vi "3. In CSM API parameters.vi"() -> ()   [LabVIEW 2017]
doc: "## Persisting CSM API Parameters (3. In CSM API parameters.vi)\n\n### Overview\n\nDemonstrates how to use the CSM INI Variable Support feature to persist parameter information in an INI configuration file.\n\n### Introduction\n\nThis example shows how to persist parameter information in an INI configuration file using CSM INI Variable Support API, primarily through `Convert API String to Cluster(Default in Session).vim` or `Convert API String to Cluster(Default in Key).vim`. They function identically to their counterparts in CSM API String Support but add the functionality of reading INI configuration files.\n\nData sources may include: information sent via message parameters, parameters in the configuration file, or default constant parameters provided at design time. They have a clear priority hierarchy: CSM API Parameters > Configuration File Parameters > Default Constant Parameters.\n\n**Notes:**\n\n- During initialization, explicitly sent parameters have the highest priority.\n- If no parameters are sent, parameters from the configuration file are used.\n- In the absence of configuration file parameters, default constant parameters are applied.\n- Parameters can be partially specified. Missing values are automatically filled using configuration information from the next priority level.\n\n### Steps\n\n- Step1: Generate a temporary INI file and load it using `CSM - Load Configuration Variables From File.vi`.\n\n- Step2: Simulate a CSM module named \"network\" using a standard loop.\n\n- Step3: Assume the passed parameter is \"ip:11.22.33.44\". This information has the highest priority and overrides the configuration in the INI file.\n\n - Step3.1: `Convert API String to Cluster(Default in Session).vim` conversion loads the key with the same name from the section. The IP information is loaded from the parameter. The port is not provided in the parameter, but port is defined as 8080 in \"network\". So the final cluster port is 8080.\n - Step3.2: `Convert API String to Cluster(Default in Session).vim` conversion loads configuration from the given section/key. The IP information is loaded from the parameter. The port is not provided in the parameter, but port is defined as 8081 in network.address1. Thus the final cluster port is 8081.\n\n- Step4: Assume the passed parameter is empty `\"\"`, equivalent to providing no parameter. In this case, the configuration from the file is prioritized.\n\n - Step4.1: `Convert API String to Cluster(Default in Session).vim` conversion loads the key with the same name from the section. The IP information uses network.ip, resulting in IP: 10.144.41.41. The port uses network.port, resulting in 8080.\n - Step4.2: `Convert API String to Cluster(Default in Session).vim` conversion loads configuration from the given section/key. Configuration is loaded from network.address1, resulting in IP:10.144.42.42 and port:8081.\n\n- Step5: Assume the passed parameter is empty `\"\"`, equivalent to providing no parameter. The corresponding configuration is not defined in the INI configuration file. In this case, default constant parameters are used.\n\n - Step5.1: `Convert API String to Cluster(Default in Session).vim` conversion. The \"non-existing module\" section does not exist, so the provided reference data is used, resulting in IP:127.0.0.1 and port:80.\n - Step5.2: `Convert API String to Cluster(Default in Session).vim` conversion. Load configuration from the given section/key, but neither exists. The provided reference data is used, resulting in IP:127.0.0.1 and port:80."
uses:
  1656162b-afee-422c-bd32-e5dc0ed47e9c.vi
  10c63860-64da-4a50-8590-83a789bccc1b.vi
  b8deca2c-73dd-4ae4-bcf2-ddb52dad5ebe.vi
  2f71b960-401c-4d78-a3a0-f07855567af6.vi
  000051f1-0e83-4b30-8694-14c2d9f7239e.vi
  0af89d8b-3541-4ee1-9e23-b806c46e6636.vi
  1656162b-afee-422c-bd32-e5dc0ed47e9c.vi/70cf541c-689a-4909-ae73-497058dc5e15.vi
  1656162b-afee-422c-bd32-e5dc0ed47e9c.vi/8441470c-f7c2-4ba6-a00e-bb382131ed64.vi
  10c63860-64da-4a50-8590-83a789bccc1b.vi/70cf541c-689a-4909-ae73-497058dc5e15.vi
  10c63860-64da-4a50-8590-83a789bccc1b.vi/9171d6c3-d5ea-4572-92dd-59f7e0660fdf.vi
  b8deca2c-73dd-4ae4-bcf2-ddb52dad5ebe.vi/70cf541c-689a-4909-ae73-497058dc5e15.vi
  b8deca2c-73dd-4ae4-bcf2-ddb52dad5ebe.vi/9171d6c3-d5ea-4572-92dd-59f7e0660fdf.vi
  2f71b960-401c-4d78-a3a0-f07855567af6.vi/70cf541c-689a-4909-ae73-497058dc5e15.vi
  2f71b960-401c-4d78-a3a0-f07855567af6.vi/8441470c-f7c2-4ba6-a00e-bb382131ed64.vi
  000051f1-0e83-4b30-8694-14c2d9f7239e.vi/70cf541c-689a-4909-ae73-497058dc5e15.vi
  000051f1-0e83-4b30-8694-14c2d9f7239e.vi/8441470c-f7c2-4ba6-a00e-bb382131ed64.vi
  0af89d8b-3541-4ee1-9e23-b806c46e6636.vi/70cf541c-689a-4909-ae73-497058dc5e15.vi
  0af89d8b-3541-4ee1-9e23-b806c46e6636.vi/9171d6c3-d5ea-4572-92dd-59f7e0660fdf.vi
  1656162b-afee-422c-bd32-e5dc0ed47e9c.vi/8441470c-f7c2-4ba6-a00e-bb382131ed64.vi/99de0c97-112a-4c86-9094-c187659127e1.vi
  <userlib>/_NEVSTOP/Communicable State Machine(CSM)/Utility/Build Error Cluster.vi
  <userlib>/_NEVSTOP/Communicable State Machine(CSM)/addons/API-String-Arugments-Support/_Support/Concatenate Strings If not Empty_csm.vi
  INI-Static-Variable-Support/_Support/FlagInstance-CSMINIVariable.vi
  2f71b960-401c-4d78-a3a0-f07855567af6.vi/8441470c-f7c2-4ba6-a00e-bb382131ed64.vi/99de0c97-112a-4c86-9094-c187659127e1.vi
  000051f1-0e83-4b30-8694-14c2d9f7239e.vi/8441470c-f7c2-4ba6-a00e-bb382131ed64.vi/99de0c97-112a-4c86-9094-c187659127e1.vi
  <userlib>/_NEVSTOP/Communicable State Machine(CSM)/_Support/ChangeFlag/ChangeFlag-Read.vi
  <userlib>/_NEVSTOP/Communicable State Machine(CSM)/_Support/ChangeFlag/ChangeFlagDB.vi
  INI-Static-Variable-Support/_Support/CSM - Read INI String.vi
  INI-Static-Variable-Support/_Support/Populate String with INI Variable.vi
  <userlib>/_NEVSTOP/Communicable State Machine(CSM)/addons/API-String-Arugments-Support/_Support/Convert API String Arguments to Data(variant).vi
  <vilib>/Utility/Data Type/Get Type Information.vi
  <userlib>/_NEVSTOP/Communicable State Machine(CSM)/addons/API-String-Arugments-Support/_Support/Data To SingleElementsArray_csm.vi
  <userlib>/_NEVSTOP/Communicable State Machine(CSM)/addons/API-String-Arugments-Support/_Support/Data To API String Arguments.vi
  INI-Static-Variable-Support/_Support/Parse Used Session and Name.vi
  INI-Static-Variable-Support/_Support/INI-FGV(lvlibp).vi
  <userlib>/_NEVSTOP/Communicable State Machine(CSM)/addons/API-String-Arugments-Support/_Support/SingleElementsArray To Data_csm.vi
  INI-Static-Variable-Support/INI-Static-Variable-Support.lvlib
panel:
  out "case1:(load from section) use default value of constant":cluster{"ip":string, "port":i32}={"ip"="127.0.0.1", "port"=80}
  out "case1:(load from key) use default value of constant":cluster{"ip":string, "port":i32}={"ip"="127.0.0.1", "port"=80}
  out "case2:(load from section) no argument, use config":cluster{"ip":string, "port":i32}={"ip"="10.144.41.41", "port"=8080}
  out "case2:(load from key) no argument, use config":cluster{"ip":string, "port":i32}={"ip"="10.144.42.42", "port"=8081}
  out "case3:(load from key) use argument value":cluster{"ip":string, "port":i32}={"ip"="11.22.33.44", "port"=8081}
  out "case3:(load from section) use argument value":cluster{"ip":string, "port":i32}={"ip"="11.22.33.44", "port"=8080}
  # "#CSM-Example overview\n\nDemonstrates how to use the CSM INI Variable Support feature to persist parameter information in an INI configuration file."
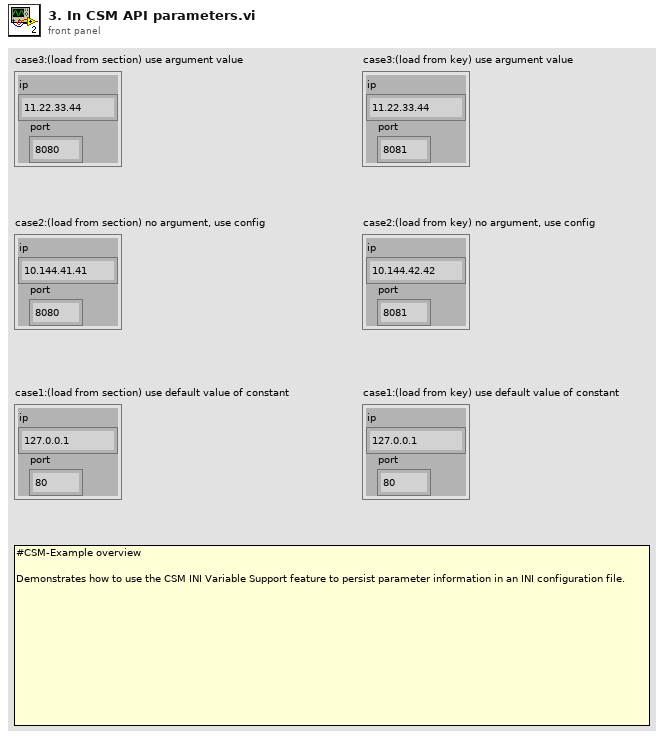
[diagram p1: front panel]
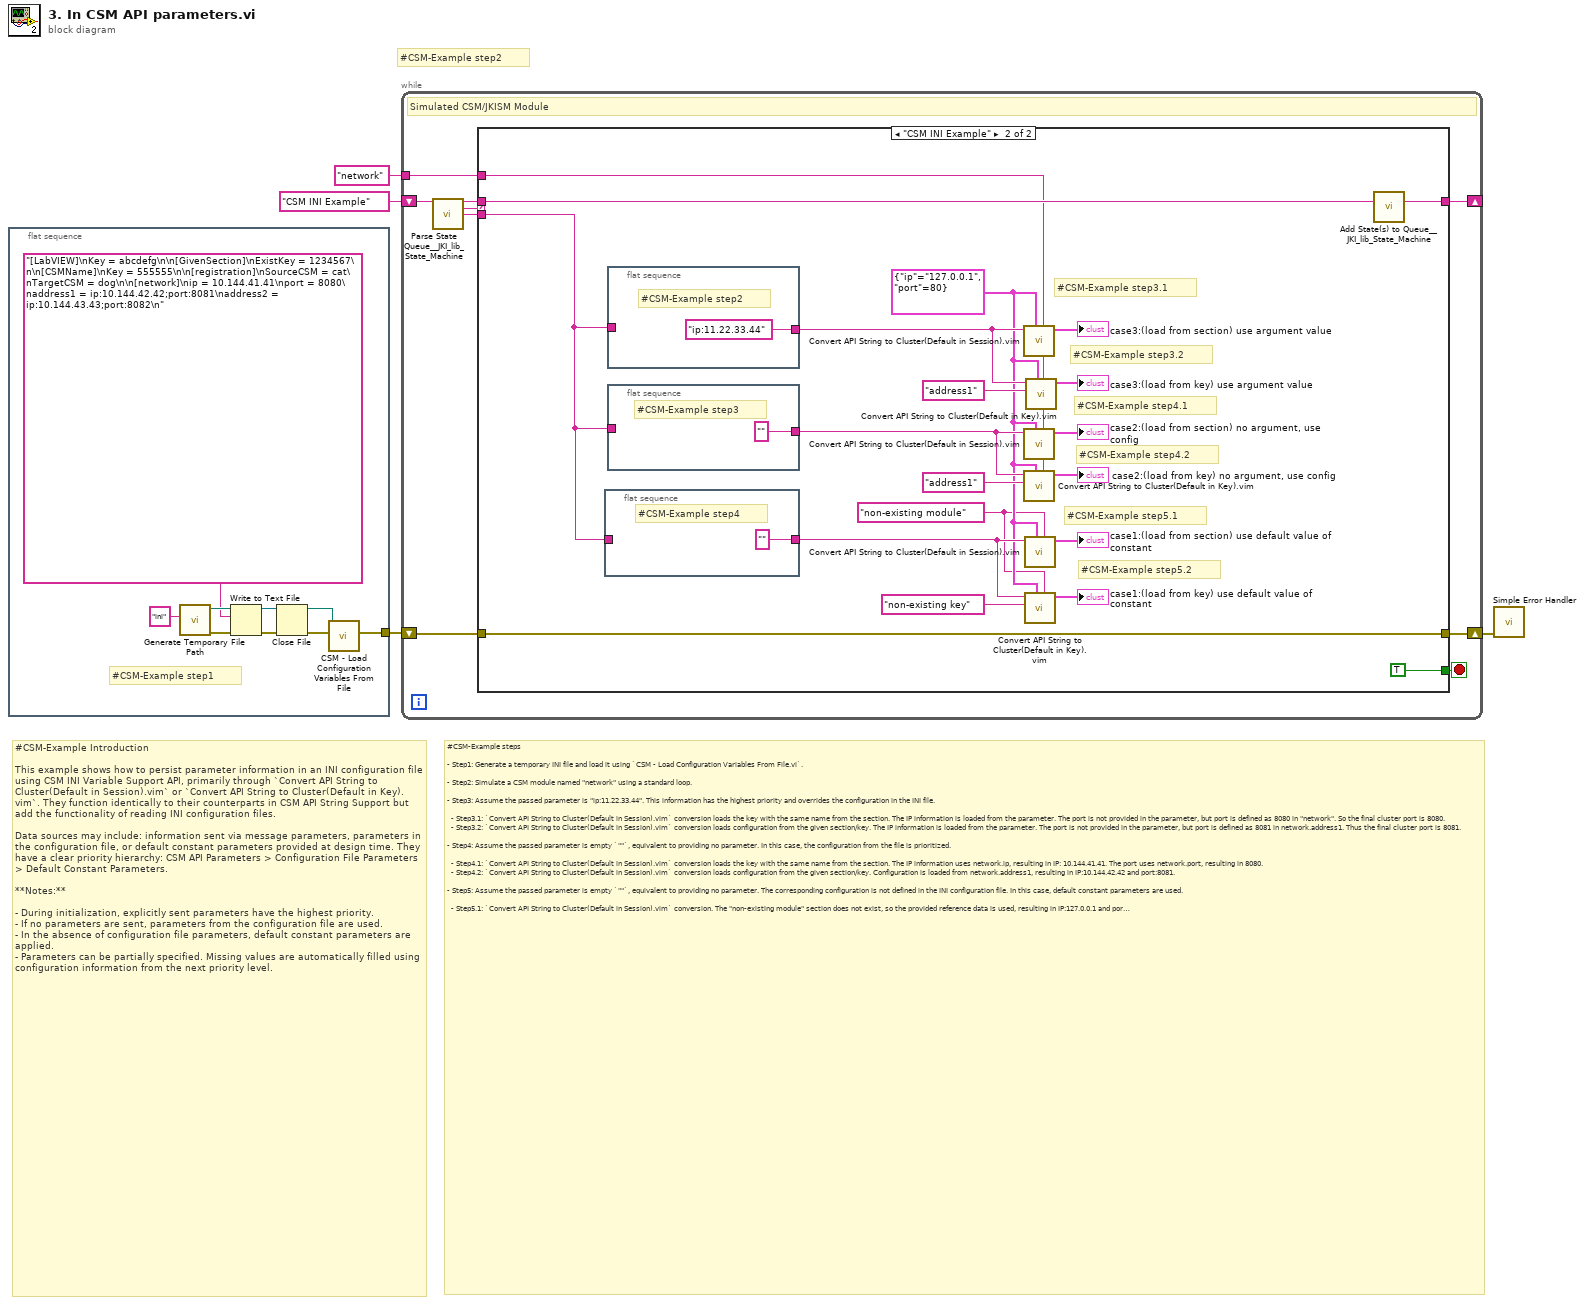
[diagram p0: block diagram]
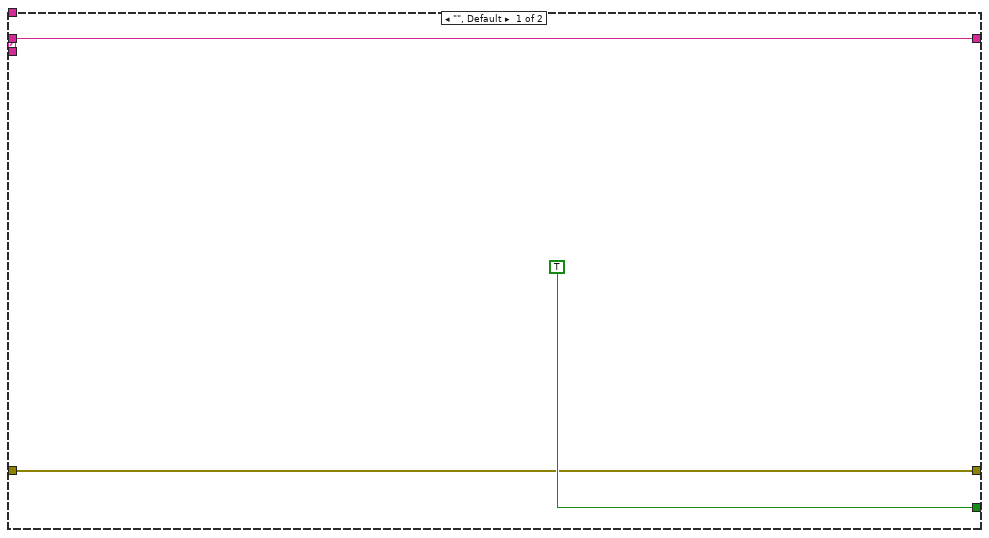
[diagram p2: hidden frame]
diagram:
  # "#CSM-Example step2"
  # "#CSM-Example steps\n\n- Step1: Generate a temporary INI file and load it using `CSM - Load Configuration Variables From File.vi`.\n\n- Step2: Simulate a CSM module named \"network\" using a standard loop.\n\n- Step3: Assume the passed parameter is \"ip:11.22.33.44\". This information has the highest priority and overrides the configuration in the INI file.\n\n  - Step3.1: `Convert API String to Cluster(Default in Session).vim` conversion loads the key with the same name from the section. The IP information is loaded from the parameter. The port is not provided in the parameter, but port is defined as 8080 in \"network\". So the final cluster port is 8080.\n  - Step3.2: `Convert API String to Cluster(Default in Session).vim` conversion loads configuration from the given section/key. The IP information is loaded from the parameter. The port is not provided in the parameter, but port is defined as 8081 in network.address1. Thus the final cluster port is 8081.\n\n- Step4: Assume the passed parameter is empty `\"\"`, equivalent to providing no parameter. In this case, the configuration from the file is prioritized.\n\n  - Step4.1: `Convert API String to Cluster(Default in Session).vim` conversion loads the key with the same name from the section. The IP information uses network.ip, resulting in IP: 10.144.41.41. The port uses network.port, resulting in 8080.\n  - Step4.2: `Convert API String to Cluster(Default in Session).vim` conversion loads configuration from the given section/key. Configuration is loaded from network.address1, resulting in IP:10.144.42.42 and port:8081.\n\n- Step5: Assume the passed parameter is empty `\"\"`, equivalent to providing no parameter. The corresponding configuration is not defined in the INI configuration file. In this case, default constant parameters are used.\n\n  - Step5.1: `Convert API String to Cluster(Default in Session).vim` conversion. The \"non-existing module\" section does not exist, so the provided reference data is used, resulting in IP:127.0.0.1 and port:80.\n  - Step5.2: `Convert API String to Cluster(Default in Session).vim` conversion. Load configuration from the given section/key, but neither exists. The provided reference data is used, resulting in IP:127.0.0.1 and port:80."
  # "#CSM-Example Introduction\n\nThis example shows how to persist parameter information in an INI configuration file using CSM INI Variable Support API, primarily through `Convert API String to Cluster(Default in Session).vim` or `Convert API String to Cluster(Default in Key).vim`. They function identically to their counterparts in CSM API String Support but add the functionality of reading INI configuration files.\n\nData sources may include: information sent via message parameters, parameters in the configuration file, or default constant parameters provided at design time. They have a clear priority hierarchy: CSM API Parameters > Configuration File Parameters > Default Constant Parameters.\n\n**Notes:**\n\n- During initialization, explicitly sent parameters have the highest priority.\n- If no parameters are sent, parameters from the configuration file are used.\n- In the absence of configuration file parameters, default constant parameters are applied.\n- Parameters can be partially specified. Missing values are automatically filled using configuration information from the next priority level."
  n1 = flat-sequence {
    tunnel: [w7] -> w2
    frame #0 {
      # "#CSM-Example step1"
      n2 = call <vilib>:"Generate Temporary File Path.vi"("Temporary File Extension (tmp)"="ini") -> ("error out"=w13:errorcluster, "Unique Temporary File Path"=w10:path)  [unwired: 9 in]
      n3 = Write to Text File(file (use dialog)=w10, text="[LabVIEW]\nKey = abcdefg\n\n[GivenSection]\nExistKey = 1234567\n\n[CSMName]\nKey = 555555\n\n[registration]\nSourceCSM = cat\nTargetCSM = dog\n\n[network]\nip = 10.144.41.41\nport = 8080\naddress1 = ip:10.144.42.42;port:8081\naddress2 = ip:10.144.43.43;port:8082\n", error in=w13) -> (refnum out=w9:refnum<file>, error out=w11:errorcluster)  [unwired: 1 in, 1 out]
      n4 = Close File(refnum=w9, error in=w11) -> (path=w5:path, error out=w8:errorcluster)
      n5 = call "CSM - Load Configuration Variables From File.vi"("error in (no error)"=w8, "Configuration Path"=w5) -> ("error out"=w7:errorcluster)  [unwired: 7 in]
    }
  }
  n6 = while "Communicable State Machine(CSM) 2025" {
    shift-right: [w20] -> _
    shift-left: "CSM INI Example" ("State Queue") -> [w22]
    shift-right: [w15] -> w1
    shift-left: w2 -> [w16]
    tunnel: "network" ("State Queue") -> [w14]
    stop <- w17 stop-if-true
    # "Simulated CSM/JKISM Module"
    n7 = call <vilib>:"Parse State Queue__JKI_lib_State_Machine.vi"("State Queue"=w22) -> ("Remaining States"=w21:string, "Current State"=w19:string, "Arguments"=w18:string)  [unwired: 12 in]
    n8 = case shown="\"CSM INI Example\"" w19 {
      tunnel: w21 -> [w25 w43]
      tunnel: [w25 w42] -> w20
      tunnel: w18 -> [_ w26]
      tunnel: [TRUE TRUE] -> w17
      tunnel: w16 -> [w23 w44]
      tunnel: [w23 w44] -> w15
      tunnel: w14 -> [_ w28]
      frame "", Default {
      }
      frame "CSM INI Example" {
        w27 = "non-existing module" ("Section Name(\"\" as Default)")
        w29 = cluster{"ip":string, "port":i32} {"ip"="127.0.0.1", "port"=80}
        # "#CSM-Example step5.2"
        # "#CSM-Example step5.1"
        # "#CSM-Example step4.2"
        # "#CSM-Example step4.1"
        # "#CSM-Example step3.2"
        # "#CSM-Example step3.1"
        n9 = flat-sequence {
          tunnel: ["" ("Arguments")] -> w30
          tunnel: w26 -> [_]
          frame #0 {
            # "#CSM-Example step4"
          }
        }
        n10 = flat-sequence {
          tunnel: w26 -> [_]
          tunnel: ["ip:11.22.33.44" ("Arguments")] -> w35
          frame #0 {
            # "#CSM-Example step2"
          }
        }
        n11 = flat-sequence {
          tunnel: ["" ("Arguments")] -> w34
          tunnel: w26 -> [_]
          frame #0 {
            # "#CSM-Example step3"
          }
        }
        n12 = call "Convert API String to Cluster(Default in Session).vim"("Section Name(\"\" as Default)"=w28, "Type"=w29, "API String"=w35) -> ("Data"=→"case3:(load from section) use argument value":cluster{"ip":string, "port":i32})  [unwired: 7 in, 1 out]
        n13 = call "Convert API String to Cluster(Default in Session).vim"("Section Name(\"\" as Default)"=w28, "Type"=w29, "API String"=w34) -> ("Data"=→"case2:(load from section) no argument, use config":cluster{"ip":string, "port":i32})  [unwired: 7 in, 1 out]
        n14 = call "Convert API String to Cluster(Default in Key).vim"("Section Name(\"\" as Default)"=w28, "Type"=w29, "Variable Name"="address1", "API String"=w34) -> ("Data"=→"case2:(load from key) no argument, use config":cluster{"ip":string, "port":i32})  [unwired: 6 in, 1 out]
        n15 = call "Convert API String to Cluster(Default in Session).vim"("Section Name(\"\" as Default)"=w27, "Type"=w29, "API String"=w30) -> ("Data"=→"case1:(load from section) use default value of constant":cluster{"ip":string, "port":i32})  [unwired: 7 in, 1 out]
        n16 = call "Convert API String to Cluster(Default in Key).vim"("Section Name(\"\" as Default)"=w27, "Type"=w29, "Variable Name"="non-existing key", "API String"=w30) -> ("Data"=→"case1:(load from key) use default value of constant":cluster{"ip":string, "port":i32})  [unwired: 6 in, 1 out]
        n17 = call "Convert API String to Cluster(Default in Key).vim"("Section Name(\"\" as Default)"=w28, "Type"=w29, "Variable Name"="address1", "API String"=w35) -> ("Data"=→"case3:(load from key) use argument value":cluster{"ip":string, "port":i32})  [unwired: 6 in, 1 out]
        n18 = call <vilib>:"Add State(s) to Queue__JKI_lib_State_Machine.vi"("State(s) in (\"\")"=w43) -> ("States Out"=w42:string)  [unwired: 14 in]
      }
    }
  }
  n19 = call <vilib>:"Simple Error Handler.vi"("error in (no error)"=w1) -> ()  [unwired: 4 in, 5 out]
